vi "setMasterPort.vi"(2 "Port":u32=11311, 3 "ROS_Master.lvclass in":refnum<class "ROS_Master.lvclass">) -> (1 "ROS_Master.lvclass out":refnum<class "ROS_Master.lvclass">)   [LabVIEW 2012, in "ROS_Master.lvclass"]
uses:
  <userlib>/ROSforLV/ROS/Code/ROS_Master/ROS_Master.lvclass
  <userlib>/ROSforLV/ROS/Code/ROS_Master/ROS_Master.lvclass/ROS_Master.ctl
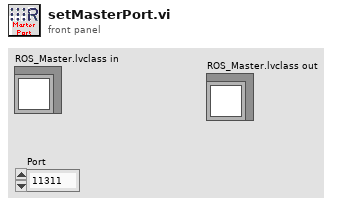
[diagram p1: front panel]
types:
  T1 = enum16{"http://IP:port", "http://IP", "IP:port", "IP only"}
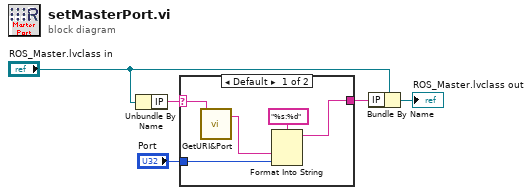
[diagram p0: block diagram]
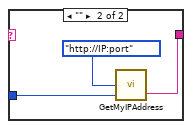
[diagram p2: hidden frame]
diagram:
  n1 = Unbundle By Name("ROS_Master.lvclass in") -> ("IP"=w5:string)
  n2 = case shown="Default" w5 {
    selector: w5 -> [w7 _]
    tunnel: [w8 w12] -> w1
    tunnel: "Port" -> [w9 w13]
    frame Default {
      n3 = call <userlib>:"GetURI&Port.vi"("URI in"=w7) -> ("URI"=w6:string)  [unwired: 1 out]
      n4 = Format Into String(format string="%s:%d", w6, w9) -> (resulting string=w8:string)  [unwired: 2 in, 1 out]
    }
    frame "" {
      n5 = call <userlib>:"GetMyIPAddress.vi"("Port"=w13, "Format"=T1."http://IP:port") -> ("URI"=w12:string)  [unwired: 2 in]
    }
  }
  n6 = Bundle By Name(cluster="ROS_Master.lvclass in", "IP"=w1) -> (→"ROS_Master.lvclass out":refnum<class "ROS_Master.lvclass">)
